vi "PUT File.vi"(6 "timeout (10000)":i32=10000, 7 "output file":path=path "", 8 "error in (no error)":errorcluster, 9 "file":path, 10 "url":string, 11 "HTTP Client Abstract in":refnum<class "HTTP Client Abstract.lvclass">) -> (0 "error out":errorcluster, 1 "body":string, 2 "headers":string, 3 "HTTP Client Abstract out":refnum<class "HTTP Client Abstract.lvclass">)   [LabVIEW 2021, in "HTTP Client Abstract.lvclass"]
uses:
  HTTP Client Abstract.lvclass
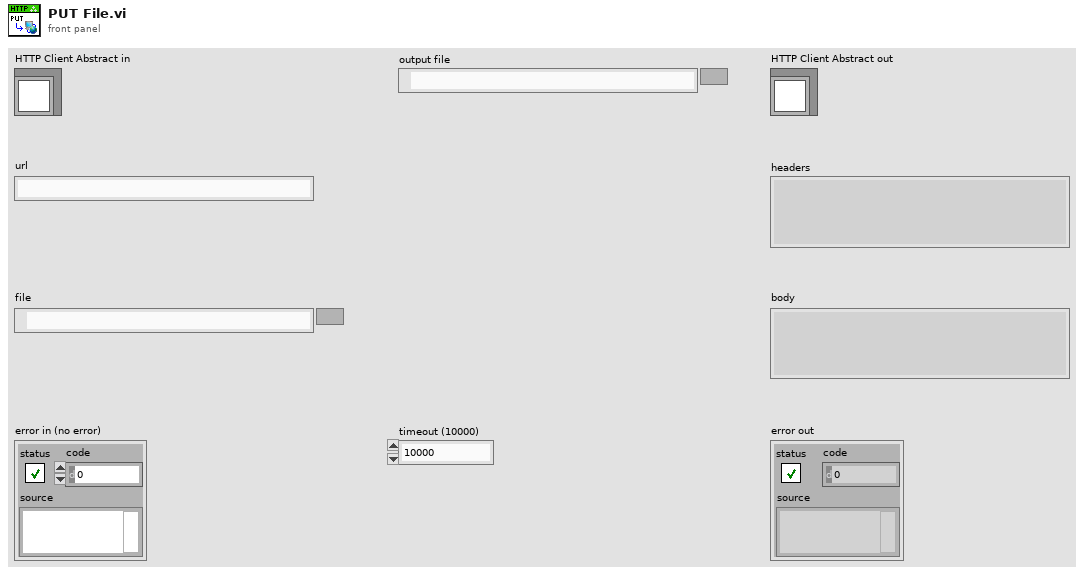
[diagram p1: front panel]
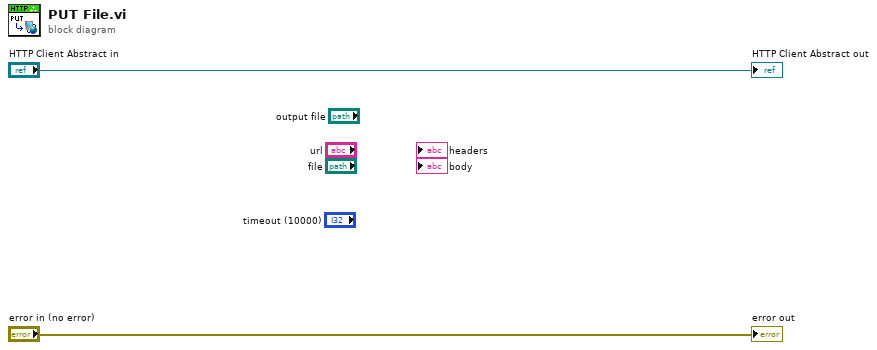
[diagram p0: block diagram]
diagram:
  "error out" <- "error in (no error)"
  "HTTP Client Abstract out" <- "HTTP Client Abstract in"
